vi "gradient_descent.vi"(4 "Gain":dbl, 5 "function data":T2, 6 "Bounds":cluster{"Minimum X":dbl[], "Maximum X":dbl[]}, 7 "objective function":T3, 8 "error in":errorcluster, 9 "stopping criteria":T1={"function tolerance"=1e-06, "parameter tolerance"=1e-06, "max iterations"=100, "max function calls"=1000, "gradient tolerance"=1e-06, "max time (sec)"=-1.0}, 11 "start":dbl[](array[numeric])) -> (0 "error out":errorcluster, 2 "f(X) min":dbl, 3 "minimum":dbl[](array[numeric]))   [LabVIEW 2013]
uses:
  <vilib>/gmath/NumericalOptimization/ucno_user objective function ref.ctl
  <vilib>/gmath/NumericalOptimization/objective function data.ctl
  <vilib>/gmath/NumericalOptimization/stopping criteria.ctl
  <vilib>/gmath/NI_Gmath.lvlib
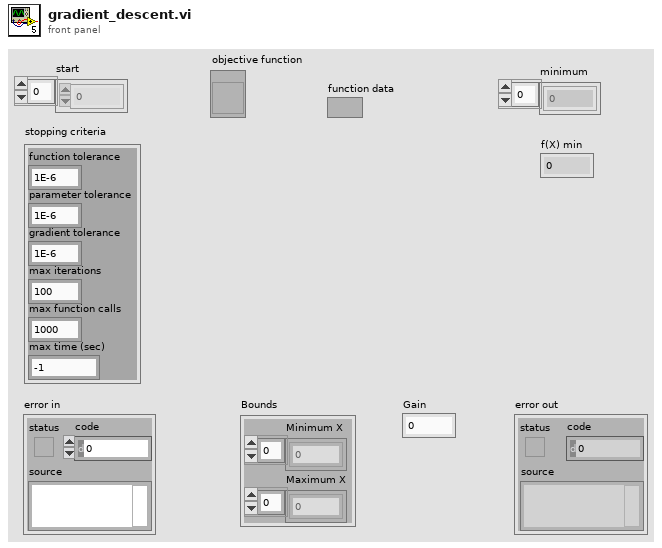
[diagram p1: front panel]
types:
  T1 = typedef "NI_Gmath.lvlib/stopping criteria.ctl" = cluster{"function tolerance":dbl, "parameter tolerance":dbl, "max iterations":i32, "max function calls":i32, "gradient tolerance":dbl, "max time (sec)":dbl}
  T2 = typedef "NI_Gmath.lvlib/objective function data.ctl" = variant
  T3 = typedef "NI_Gmath.lvlib/ucno_user objective function ref.ctl" = refnum<vi>
  T4 = cluster{"objective function":bool, "gradient":bool}
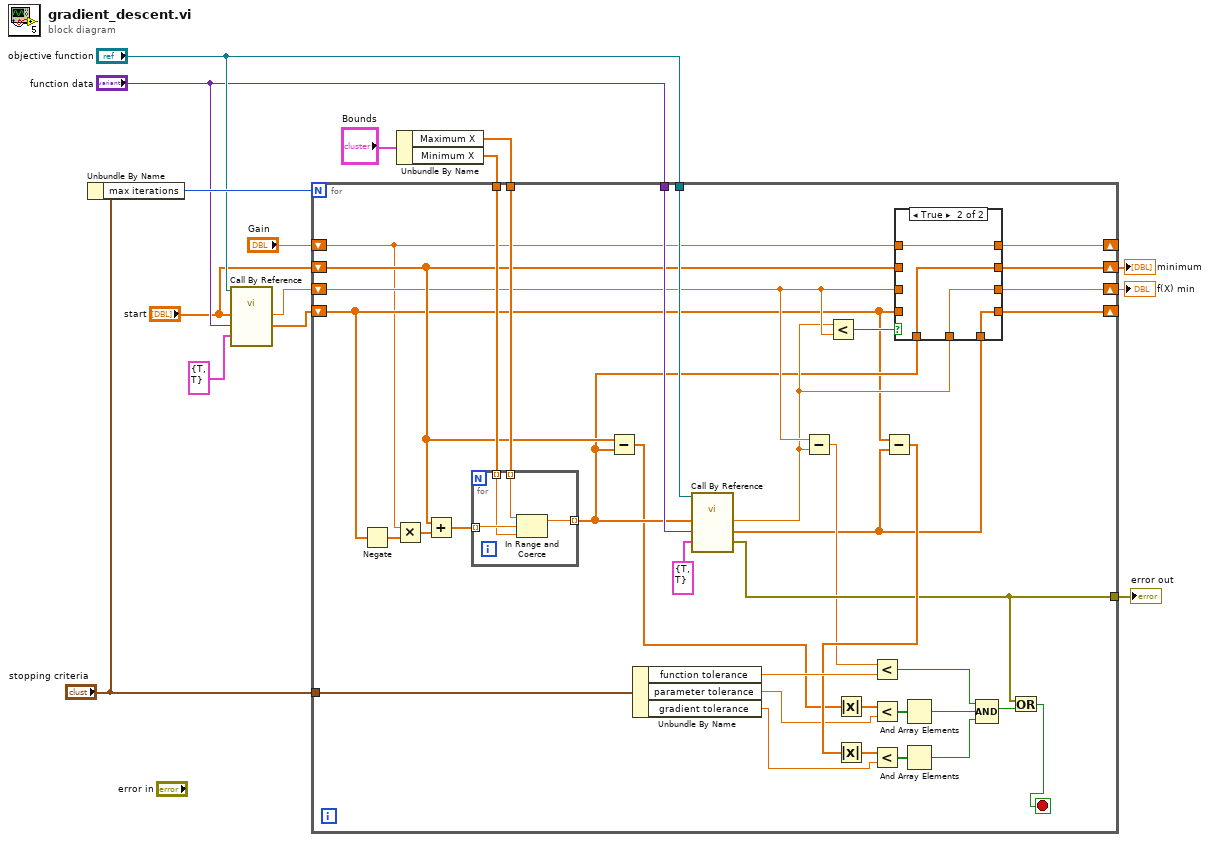
[diagram p0: block diagram]
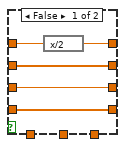
[diagram p2: hidden frame]
diagram:
  n1 = Unbundle By Name("stopping criteria") -> ("max iterations"=w14:i32)
  n2 = call-by-ref "?"(reference="objective function", "output control"=T4 {"objective function"=TRUE, "gradient"=TRUE}, "data"="function data", "X"="start") -> ("gradient"=w12:dbl[], "f(X)"=w3:dbl)  [unwired: 1 in, 3 out]
  n3 = Unbundle By Name("Bounds") -> ("Maximum X"=w7:dbl[], "Minimum X"=w6:dbl[])
  n4 = for {
    N: w14 -> [_]
    tunnel: [w32] -> w15
    tunnel: "stopping criteria" -> [w51]
    shift-right: [w24] -> w2
    shift-left: "start" -> [w28]
    shift-right: [w22] -> _
    shift-left: w12 -> [w20]
    shift-right: [w25] -> w1
    shift-left: w3 -> [w27]
    tunnel: "objective function" -> [w50]
    tunnel: "function data" -> [w49]
    tunnel: w7 -> [w45]
    tunnel: w6 -> [w44]
    shift-right: [w19] -> _
    shift-left: "Gain" -> [w18]
    stop <- w31 stop-if-true
    n5 = Negate(x=w20) -> (-x=w48:dbl[])
    n6 = Multiply(x=w18, y=w48) -> (x*y=w47:dbl[])
    n7 = Add(x=w28, y=w47) -> (x+y=w46:dbl[])
    n8 = for {
      tunnel: w46 -> [w65] mode=indexing
      tunnel: [w64] -> w23 mode=indexing
      tunnel: w45 -> [w63] mode=indexing
      tunnel: w44 -> [w62] mode=indexing
      n9 = In Range and Coerce(upper limit=w63, x=w65, lower limit=w62) -> (coerced(x)=w64:dbl)  [unwired: 1 out]
    }
    n10 = Subtract(x=w28, y=w23) -> (x-y=w17:dbl[])
    n11 = Unbundle By Name(w51) -> ("function tolerance"=w43:dbl, "parameter tolerance"=w16:dbl, "gradient tolerance"=w37:dbl)
    n12 = call-by-ref "?"(reference=w50, "output control"=T4 {"objective function"=TRUE, "gradient"=TRUE}, "data"=w49, "X"=w23) -> ("error out"=w32:errorcluster, "gradient"=w21:dbl[], "f(X)"=w26:dbl)  [unwired: 1 in, 2 out]
    n13 = Subtract(x=w27, y=w26) -> (x-y=w30:dbl)
    n14 = Less?(x=w26, y=w27) -> (x < y?=w29:bool)
    n15 = Absolute Value(x=w17) -> (abs(x)=w42:dbl[])
    n16 = Less?(x=w30, y=w43) -> (x < y?=w36:bool)
    n17 = Less?(x=w42, y=w16) -> (x < y?=w41:bool[])
    n18 = Subtract(x=w20, y=w21) -> (x-y=w38:dbl[])
    n19 = Absolute Value(x=w38) -> (abs(x)=w39:dbl[])
    n20 = Less?(x=w39, y=w37) -> (x < y?=w40:bool[])
    n21 = case shown="True" w29 {
      tunnel: w28 -> [w57 _]
      tunnel: w27 -> [w56 _]
      tunnel: [w57 w61] -> w24
      tunnel: w23 -> [_ w61]
      tunnel: w26 -> [_ w60]
      tunnel: [w56 w60] -> w25
      tunnel: [w55 w59] -> w22
      tunnel: w21 -> [_ w59]
      tunnel: w20 -> [w55 _]
      tunnel: [w53 w58] -> w19
      tunnel: w18 -> [w54 w58]
      frame False {
        n22 = expression code="x/2"(w54) -> (w53:dbl)
      }
      frame True {
      }
    }
    n23 = And Array Elements(Boolean array=w41) -> (logical AND=w35:bool)
    n24 = And Array Elements(Boolean array=w40) -> (logical AND=w34:bool)
    n25 = Compound Arithmetic op=AND(w36, w35, w34) -> (w33:bool)
    n26 = Or(x=w32, y=w33) -> (x .or. y?=w31:bool)
  }
  "minimum" <- w2
  "error out" <- w15
  "f(X) min" <- w1
